vi "StepEditInterface.vi"() -> ()   [LabVIEW 2014]
panel:
  in  "ProjectList":i32(listbox)
  in  "StepList":i32(listbox)
  in  "ModifyStep":bool
  in  "RemoveStep":bool
  in  "AddStep":bool
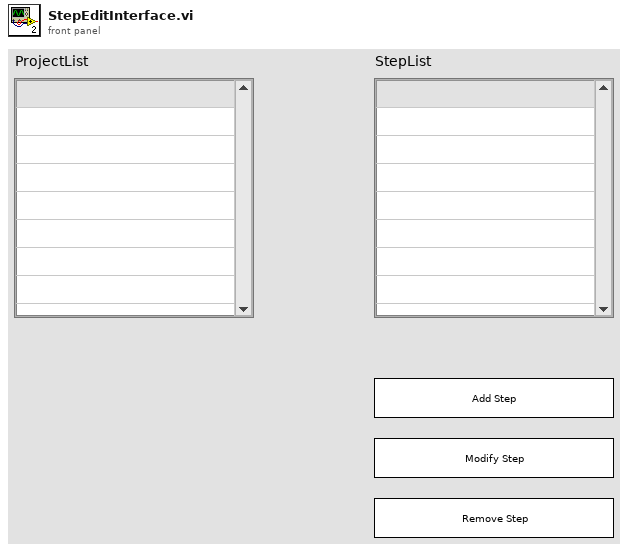
[diagram p1: front panel]
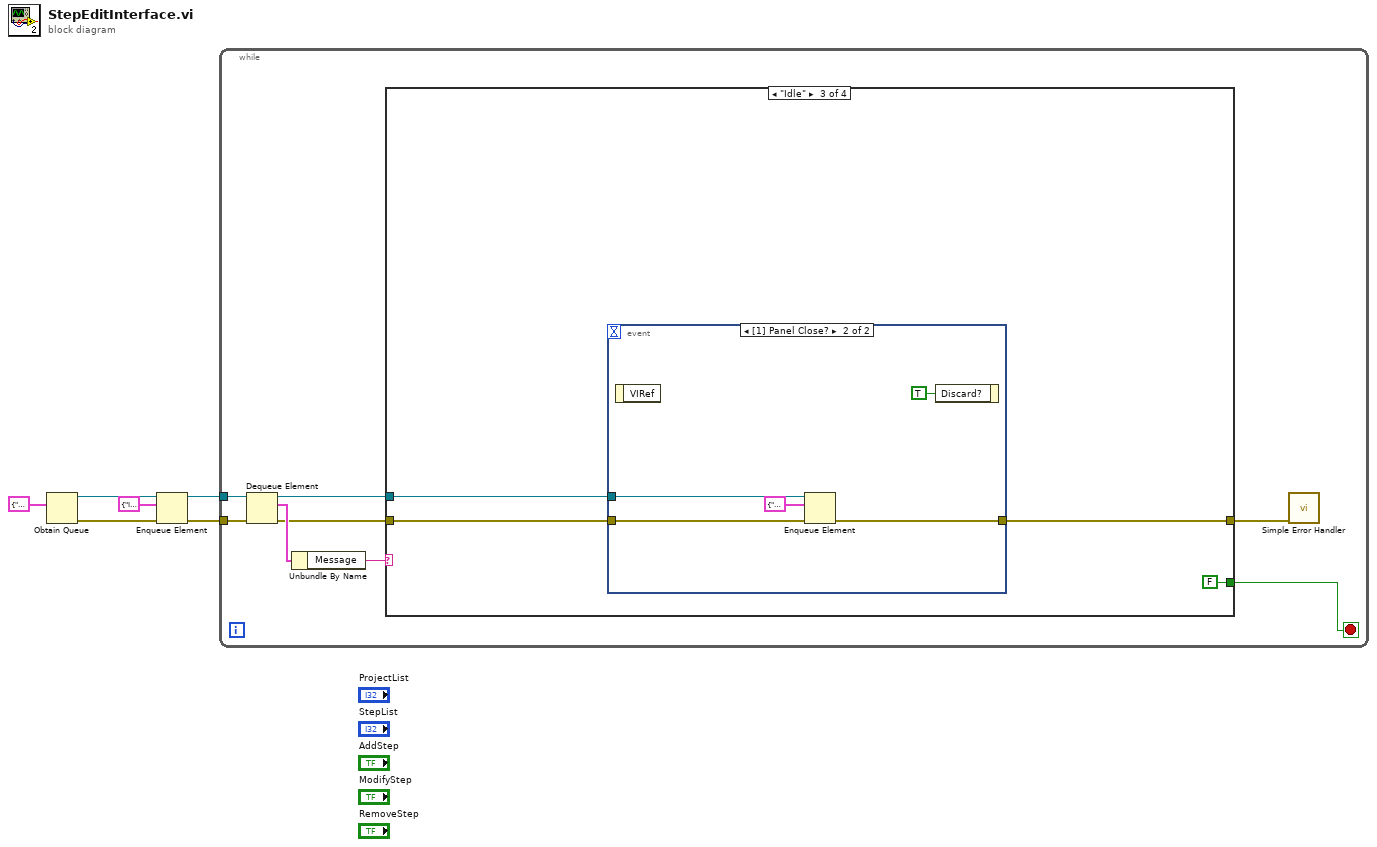
[diagram p0: block diagram]
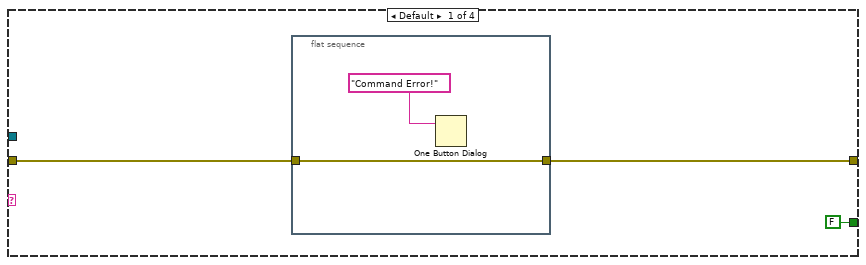
[diagram p2: hidden frame]
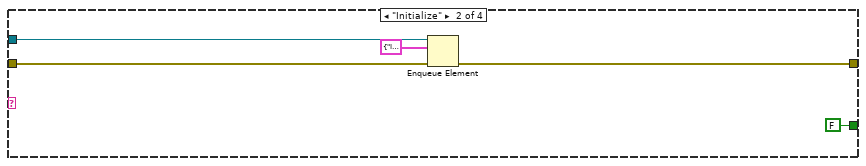
[diagram p3: hidden frame]
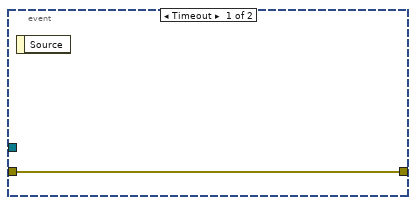
[diagram p4: hidden frame]
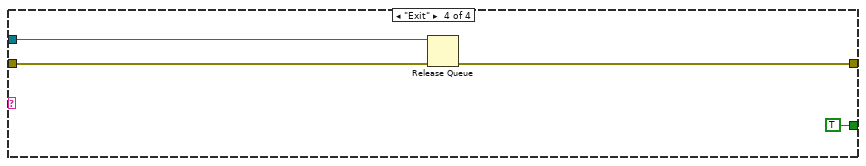
[diagram p5: hidden frame]
diagram:
  n1 = Obtain Queue(element data type=cluster{"Message":string, "Data":variant} {"Message"="", "Data"=variant}) -> (queue out=w5:refnum<queue>, error out=w6:errorcluster)  [unwired: 4 in, 1 out]
  n2 = Enqueue Element(queue=w5, element=cluster{"Message":string, "Data":variant} {"Message"="Initialize", "Data"=variant}, error in (no error)=w6) -> (queue out=w2:refnum<queue>, error out=w1:errorcluster)  [unwired: 1 in, 1 out]
  n3 = while {
    tunnel: w2 -> [w14]
    tunnel: w1 -> [w13]
    stop <- w7 stop-if-true
    n4 = Dequeue Element(queue=w14, error in (no error)=w13) -> (queue out=w8:refnum<queue>, element=w12:cluster{"Message":string, "Data":variant}, error out=w10:errorcluster)  [unwired: 1 in, 1 out]
    n5 = Unbundle By Name(w12) -> ("Message"=w11:string)
    n6 = case shown="\"Idle\"" w11 {
      tunnel: w10 -> [w17 w24 w27 w37]
      tunnel: [w16 w23 w26 w35] -> w9
      tunnel: w8 -> [_ w22 w28 w36]
      tunnel: [FALSE FALSE FALSE TRUE] -> w7
      frame Default {
        n7 = flat-sequence {
          tunnel: w17 -> [w19]
          tunnel: [w19] -> w16
          frame #0 {
            n8 = One Button Dialog(message="Command Error!") -> ()  [unwired: 1 in, 1 out]
          }
        }
      }
      frame "Initialize" {
        n9 = Enqueue Element(queue=w22, element=cluster{"Message":string, "Data":variant} {"Message"="Idle", "Data"=variant}, error in (no error)=w24) -> (error out=w23:errorcluster)  [unwired: 1 in, 2 out]
      }
      frame "Idle" {
        n10 = event shown="[1] Panel Close?" {
          selector: _ -> [_ _]
          dyn-events: _ -> [_ _]
          timeout: _ -> [_ _]
          tunnel: w28 -> [_ w31]
          tunnel: w27 -> [w29 w33]
          tunnel: [w29 w32] -> w26
          event Timeout {
            n11 = event-data() -> ()  [unwired: 1 in, 1 out]
          }
          event Panel Close? {
            n12 = event-data() -> ()  [unwired: 1 in, 1 out]
            n13 = Enqueue Element(queue=w31, element=cluster{"Message":string, "Data":variant} {"Message"="Exit", "Data"=variant}, error in (no error)=w33) -> (error out=w32:errorcluster)  [unwired: 1 in, 2 out]
            n14 = event-data("Discard?"=TRUE) -> ()  [unwired: 1 in, 1 out]
          }
        }
      }
      frame "Exit" {
        n15 = Release Queue(queue=w36, error in (no error)=w37) -> (error out=w35:errorcluster)  [unwired: 1 in, 2 out]
      }
    }
    n16 = call <vilib>:"Simple Error Handler.vi"("error in (no error)"=w9) -> ()  [unwired: 4 in, 5 out]
  }
